vi "Bertta_v09_7.vi"() -> ()   [LabVIEW 2015]
panel:
  out "element":bool
  out "Started:":string
  in  "SHUTDOWN":bool
  in  "MASTER CONTROL":bool
  in  "Tab Control":T1(tab)
  in  "Read Seq":bool
  in  "Save Seq":bool
  in  "Configuration file":path=path "C:/Users/shresplab/Desktop/BerttaConfiguration.lvm" caption="Filename"
  in  "OK Button 2":bool
  out "Boolean":bool
  in  "User (initials)":string
  in  "Project name":string
  in  "Description":string
  out "Output file":string
  out "PUMP1":bool
  out "Target amount":dbl
  out "Scale weight":dbl
  out "Amount now":dbl
  out "Flow rate":dbl
  out "Time to target":dbl format="%<%H:%M:%S>t"
  out "Current step":dbl
  out "Target":dbl
  out "Amount now":dbl
  out "Amount now":dbl
  out "Target":dbl
  out "Current step":dbl
  out "Time to target":dbl format="%<%H:%M:%S>t"
  out "Flow rate":dbl
  out "Amount now":dbl
  out "Scale weight":dbl
  out "Target amount":dbl
  out "PUMP2":bool
  out "Sensor OK 6":bool
  out "Sensor OK 5":bool
  out "Sensor OK 4":bool
  out "Sensor OK 3":bool
  in  "OK Button":bool
  in  "Add comment":string
  out "PUMP3":bool
  out "Target amount":dbl
  out "Scale weight":dbl
  out "Amount now":dbl
  out "Flow rate":dbl
  out "Time to target":dbl format="%<%H:%M:%S>t"
  out "Current step":dbl
  out "Target":dbl
  out "Amount now":dbl
  out "Tr":dbl
  out "Tj in":dbl
  out "Tj out":dbl
  out "T set":dbl
  out "Current step":i32
  out "RPM":dbl
  out "Torque 2":dbl
  out "Waveform Chart 5":dynamicdata(graph)
  out "Waveform Chart 6":dynamicdata(graph)
  out "Waveform Chart 7":dynamicdata(graph)
  in  "Tab Control 2":T2(tab)
  out "Waveform Chart 3":dynamicdata(graph)
  out "Waveform Chart 8":dynamicdata(graph)
  out "Waveform Chart 11":dynamicdata(graph)
  out "Waveform Chart 13":dynamicdata(graph)
  out "Waveform Chart 9":dynamicdata(graph)
  out "Table":string[][](table)=[["14.8.2017 18.06.59", "0,000000", "417,670000", "-0,150000", "1,000000", "22,220000", "23,366837", "23,574959", "23,985852", "23,690000", "240,000000", "4,000000", "0,000000", "397,000000", "-397,000000", "1,000000"], ["14.8.2017 18.07.06", "0,000000", "417,640000", "-0,120000", "1,000000", "22,220000", "23,763115", "23,906257", "23,985694", "23,680000", "240,000000", "4,000000", "0,000000", "397,000000", "-397,000000", "1,000000"], ["14.8.2017 18.07.13", "0,000000", "417,640000", "-0,120000", "1,000000", "22,220000", "23,965922", "24,013440", "23,984906", "23,670000", "240,000000", "4,100000", "3,000000", "397,000000", "-397,000000", "1,000000"], ["14.8.2017 18.07.21", "0,000000", "417,640000", "-0,120000", "1,000000", "22,220000", "23,943860", "23,900110", "23,987113", "23,670000", "240,000000", "4,000000", "0,000000", "397,000000", "-397,000000", "1,000000"], ["14.8.2017 18.07.28", "0,000000", "417,640000", "-0,120000", "1,000000", "22,220000", "23,736328", "23,600018", "23,989004", "23,660000", "240,000000", "4,000000", "0,000000", "397,000000", "-397,000000", "1,000000"], ["14.8.2017 18.07.36", "0,000000", "417,640000", "-0,120000", "1,000000", "22,220000", "23,480910", "23,324538", "23,991053", "23,660000", "240,000000", "4,000000", "0,000000", "397,000000", "-397,000000", "1,000000"], ["14.8.2017 18.07.43", "0,000000", "417,640000", "-0,120000", "2,000000", "22,220000", "23,195579", "23,008270", "23,999093", "23,650000", "240,000000", "4,000000", "0,000000", "397,000000", "-397,000000", "1,000000"], ["14.8.2017 18.07.51", "0,000000", "417,650000", "-417,650000", "1,000000", "22,220000", "22,862541", "22,649021", "24,003979", "23,650000", "240,000000", "4,000000", "0,000000", "397,000000", "-397,000000", "2,000000"], ["14.8.2017 18.07.58", "0,000000", "417,640000", "0,010000", "1,000000", "22,220000", "22,541353", "22,354878", "24,005398", "23,650000", "240,000000", "4,000000", "0,000000", "397,000000", "-397,000000", "1,000000"], ["14.8.2017 18.08.06", "0,000000", "417,640000", "0,010000", "1,000000", "22,220000", "22,347931", "22,253738", "24,007605", "23,640000", "240,000000", "4,100000", "0,000000", "397,000000", "-397,000000", "1,000000"], ["14.8.2017 18.08.13", "0,000000", "417,640000", "0,010000", "1,000000", "22,220000", "22,329030", "22,302102", "24,006028", "23,640000", "240,000000", "4,000000", "0,000000", "395,820000", "-395,820000", "1,000000"], ["14.8.2017 18.08.20", "0,000000", "417,640000", "0,010000", "1,000000", "22,220000", "22,466849", "22,511320", "24,002403", "23,630000", "240,000000", "4,000000", "0,000000", "395,830000", "-0,010000", "1,000000"], ["14.8.2017 18.08.28", "0,000000", "417,640000", "0,010000", "1,000000", "22,220000", "22,707062", "22,835101", "24,000984", "23,620000", "240,000000", "4,000000", "0,000000", "395,830000", "-0,010000", "1,000000"], ["14.8.2017 18.08.35", "0,000000", "417,640000", "0,010000", "1,000000", "22,220000", "23,054104", "23,232979", "24,001299", "23,600000", "240,000000", "4,000000", "0,000000", "395,830000", "-0,010000", "1,000000"], ["14.8.2017 18.08.43", "0,000000", "417,640000", "0,010000", "1,000000", "22,220000", "23,412371", "23,522793", "24,002560", "23,590000", "240,000000", "4,000000", "0,000000", "395,820000", "0,000000", "1,000000"], ["14.8.2017 18.08.51", "0,000000", "417,640000", "0,010000", "1,000000", "22,220000", "23,596247", "23,656125", "24,003821", "23,580000", "240,000000", "4,000000", "0,000000", "395,820000", "0,000000", "1,000000"]]
  in  "Reset":bool
  in  "Numeric 4":dbl=20.0
  in  "Numeric 3":dbl=30.0
  in  "Numeric 2":dbl=40.0
  in  "Numeric 1":dbl=30.0
  in  "Numeric":dbl=20.0
  out "Boolean 12":bool
  out "Boolean 7":bool
  out "Boolean 6":bool
  out "Boolean 5":bool
  out "Boolean 4":bool
  out "Boolean 19":bool
  in  "Numeric 5":dbl=5.0
  in  "Numeric 6":dbl=5.0
  in  "Numeric 7":dbl=5.0
  in  "Numeric 8":dbl=5.0
  in  "T ext / T ext 2":enum32{"External 1", "External 2"}(radio)
  out "Sensor OK":bool
  in  "T fail":dbl=20.0
  in  "?":bool
  in  "T manual setpoint":dbl=20.0
  in  "Lauda port":dbl=9.0
  in  "Manual select":enum32{"Tr", "Tj"}(radio)
  in  "PAUSE":bool
  out "Waveform Chart":dynamicdata(graph)
  out "T external 2":dbl
  out "Led11 5":bool
  in  "Port":i32=10
  in  "Radio Buttons 4":enum32{"Reglo Digital", "Reglo Analog", "PAM"}(radio)
  out "Speed":dbl
  out "mA":dbl format="%#_2g"
  in  "Port":i32=16
  out "RPM":dbl format="%_4f"
  out "Led10 3":bool
  out "Led9 3":bool
  out "Led8 3":bool
  out "Led7 3":bool
  out "Led6 3":bool
  out "Led5 3":bool
  out "Led4 3":bool
  out "Led3 3":bool
  out "Led2 3":bool
  out "Led1 3":bool
  in  "PumpSeq 4":dbl[][](array[numeric])=[[1.0, 2.0, 0.0], [2.0, 2.0, 0.0], [3.0, 2.0, 0.0], [0.0, 0.0, 0.0], [0.0, 0.0, 0.0], [0.0, 0.0, 0.0], [0.0, 0.0, 0.0], [0.0, 0.0, 0.0], [0.0, 0.0, 0.0], [0.0, 0.0, 0.0], [0.0, 1.0, 0.0]]
  in  "?":bool
  out "Flow rate (g/min)":dbl
  out "Scale reading":dbl
  out "Step amount now":dbl
  in  "Grams / min":dbl
  out "Waveform Chart 14":dynamicdata(graph)
  in  "?":bool
  out "Total amount now":dbl
  out "Led11 4":bool
  in  "Reset 5":bool
  out "Elapsed / step":i32
  out "Time to target":dbl format="%<%H:%M:%S>t"
  out "Led11":bool
  in  "Port":i32=11
  in  "Radio Buttons 2":enum32{"Reglo Digital", "Reglo Analog", "PAM"}(radio)
  out "Speed":dbl
  out "mA":dbl format="%#_2g"
  in  "Port":i32=15
  out "RPM":dbl format="%_4f"
  out "Led10":bool
  out "Led9":bool
  out "Led8":bool
  out "Led7":bool
  out "Led6":bool
  out "Led5":bool
  out "Led4":bool
  out "Led3":bool
  out "Led2":bool
  out "Led1":bool
  in  "PumpSeq 2":dbl[][](array[numeric])=[[1.0, 1.0, 7.0], [2.0, 1.0, 2.0], [3.0, 1.0, 100.0], [0.0, 0.0, 0.0], [0.0, 0.0, 0.0], [0.0, 0.0, 0.0], [0.0, 0.0, 0.0], [0.0, 0.0, 0.0], [0.0, 0.0, 0.0], [0.0, 0.0, 0.0], [0.0, 1.0, 0.0]]
  in  "?":bool
  out "Flow rate (g/min)":dbl
  out "Scale reading":dbl
  out "Step amount now":dbl
  in  "Grams / min":dbl
  out "Waveform Chart 10":dynamicdata(graph)
  in  "?":bool
  out "Total amount now":dbl
  out "Led11":bool
  in  "Reset 3":bool
  out "Elapsed / step":i32
  out "Time to target":dbl format="%<%H:%M:%S>t"
  out "Led11 3":bool
  in  "Port":i32=12
  in  "Radio Buttons 3":enum32{"Reglo Digital", "Reglo Analog", "PAM"}(radio)
  out "Speed":dbl
  out "mA":dbl format="%#_2g"
  in  "Port":i32=14
  out "RPM":dbl format="%_4f"
  out "Led10 2":bool
  out "Led9 2":bool
  out "Led8 2":bool
  out "Led7 2":bool
  out "Led6 2":bool
  out "Led5 2":bool
  out "Led4 2":bool
  out "Led3 2":bool
  out "Led2 2":bool
  out "Led1 2":bool
  in  "PumpSeq 3":dbl[][](array[numeric])=[[1.0, 1.0, 7.0], [2.0, 1.0, 2.0], [3.0, 1.0, 100.0], [0.0, 0.0, 0.0], [0.0, 0.0, 0.0], [0.0, 0.0, 0.0], [0.0, 0.0, 0.0], [0.0, 0.0, 0.0], [0.0, 0.0, 0.0], [0.0, 0.0, 0.0], [0.0, 1.0, 0.0]]
  in  "?":bool
  out "Flow rate (g/min)":dbl
  out "Scale reading":dbl
  out "Step amount now":dbl
  in  "Grams / min":dbl
  out "Waveform Chart 12":dynamicdata(graph)
  in  "?":bool
  out "Total amount now":dbl
  out "Led11 2":bool
  in  "Reset 4":bool
  out "Elapsed / step":i32
  out "Time to target":dbl format="%<%H:%M:%S>t"
  in  "Bypass select 2":enum32{"Remote", "Manual"}(radio)=enum."Manual"
  in  "Port":dbl=13.0
  out "RPM":dbl
  out "Torque":dbl
  in  "Set RPM":dbl(slide) scale=0.0..2000.0
  out "Waveform Chart 4":dynamicdata(graph)
  in  "Treshold (T/C)":dbl=0.5
  out "DAQ 9217 (PT100)":errorcluster
  out "Config File":dbl[][](array[numeric])
  # "Temperature sensor:"
  # "Manual control:"
  # "PUMP & SCALE 1"
  # "STEP"
  # "TOTAL"
  # "PUMP & SCALE 2"
  # "STEP"
  # "TOTAL"
  # "PUMP & SCALE 3"
  # "STEP"
  # "TOTAL"
  # "Manual control"
  # "Secondary temperature sensor"
  # "Device communication"
  # "Temp"
  # "Time"
  # "Grams    /   min"
  # "End of sequence"
  # "Manual control"
  # "Device communication"
  # "Pump configuration"
  # "Scale configuration"
  # "SCALE 1"
  # "Grams    /   min"
  # "End of sequence"
  # "Manual control"
  # "Device communication"
  # "Pump configuration"
  # "Scale configuration"
  # "SCALE 2"
  # "Grams    /   min"
  # "End of sequence"
  # "Manual control"
  # "Device communication"
  # "Pump configuration"
  # "Scale configuration"
  # "SCALE 3"
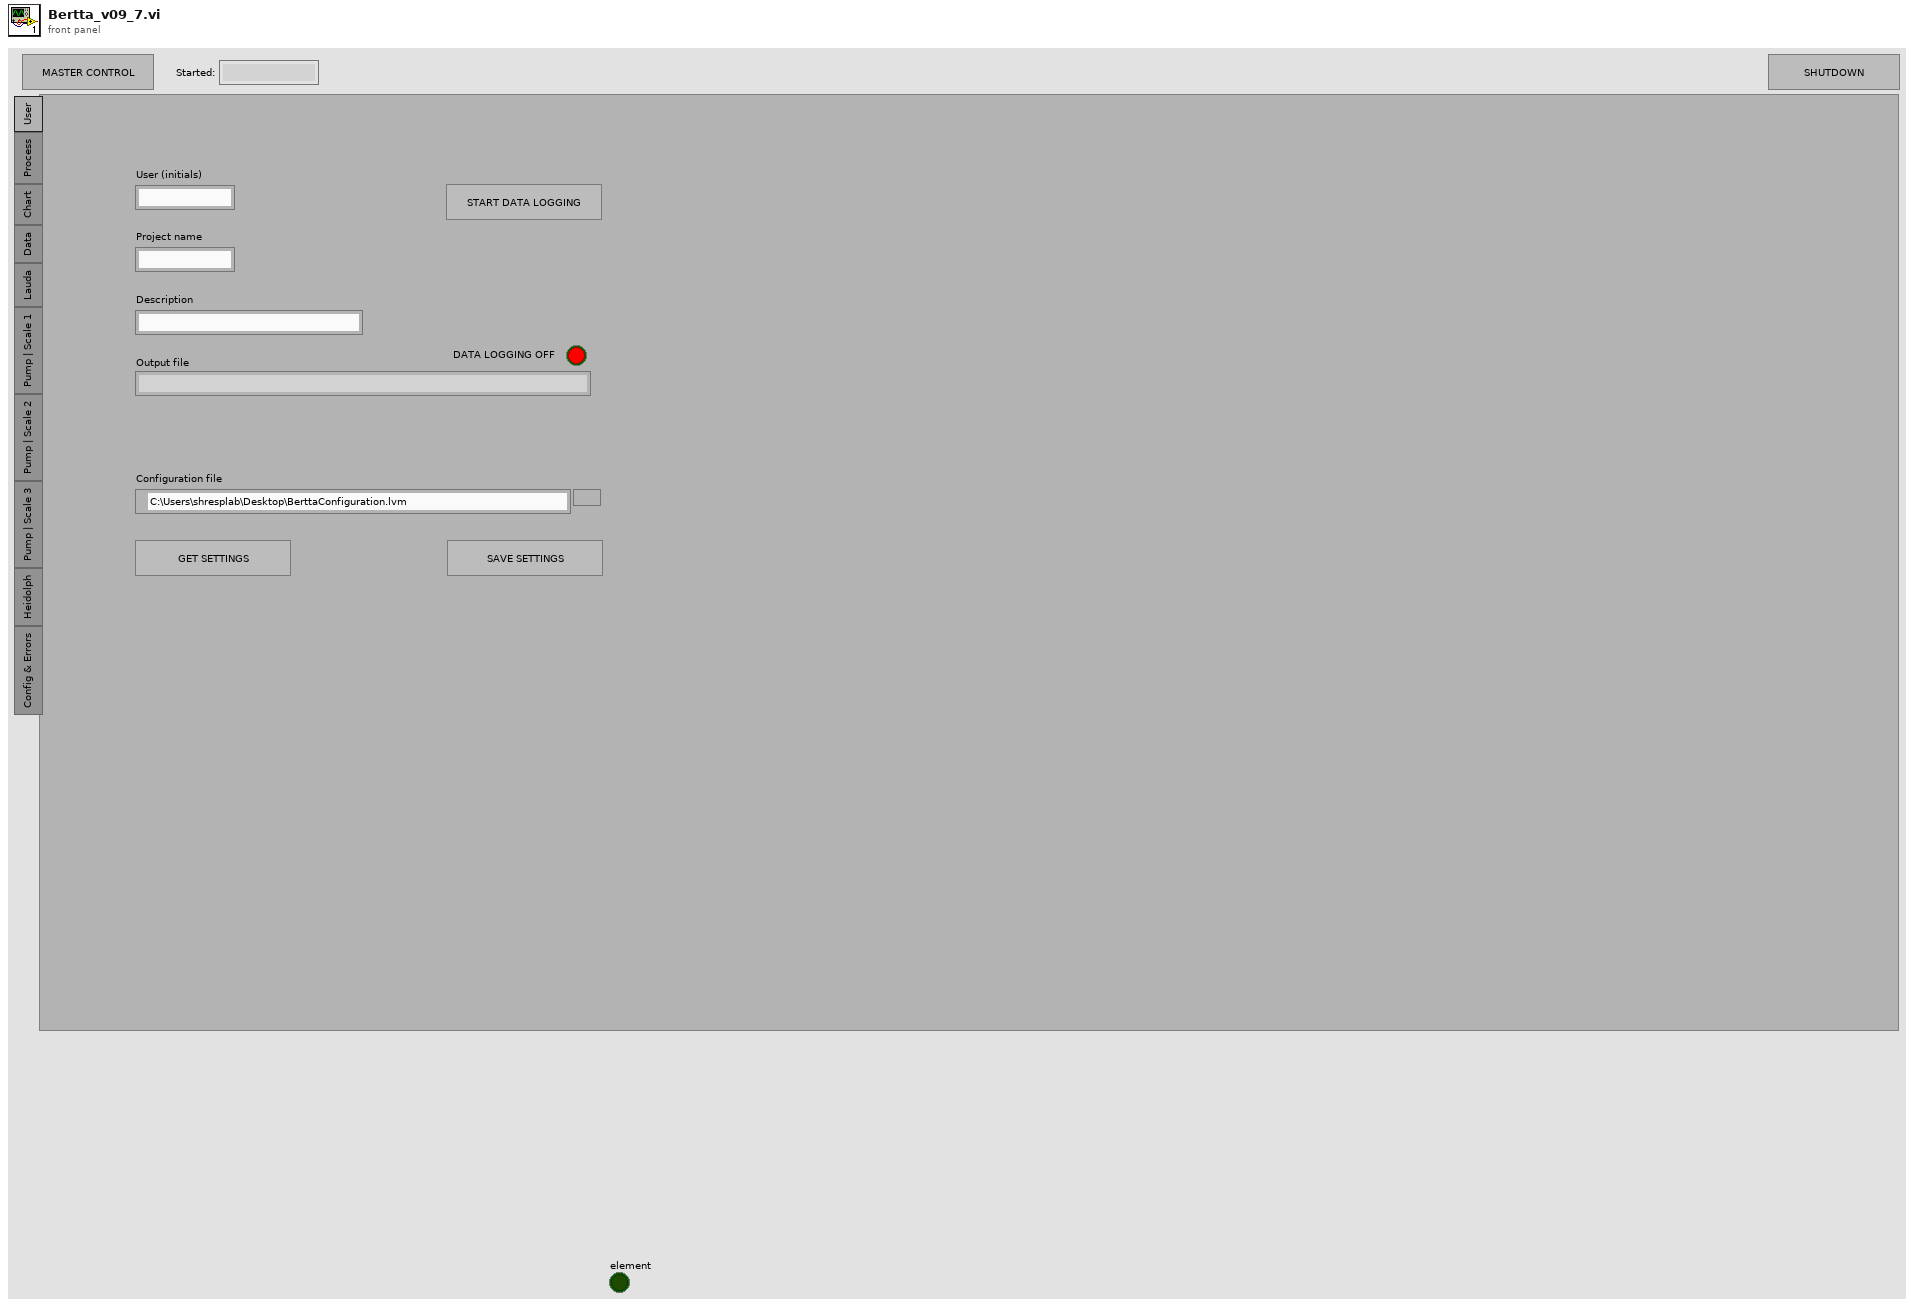
[diagram p1: front panel]
types:
  T1 = enum32{"User", "Process", "Chart", "Data", "Lauda", "Pump | Scale 1", "Pump | Scale 2", "Pump | Scale 3", "Heidolph", "Config & Errors"}
  T2 = enum32{"Temperatures", "Scale / Pump 1", "Scale / Pump 2", "Scale / Pump 3", "RPM / torque"}
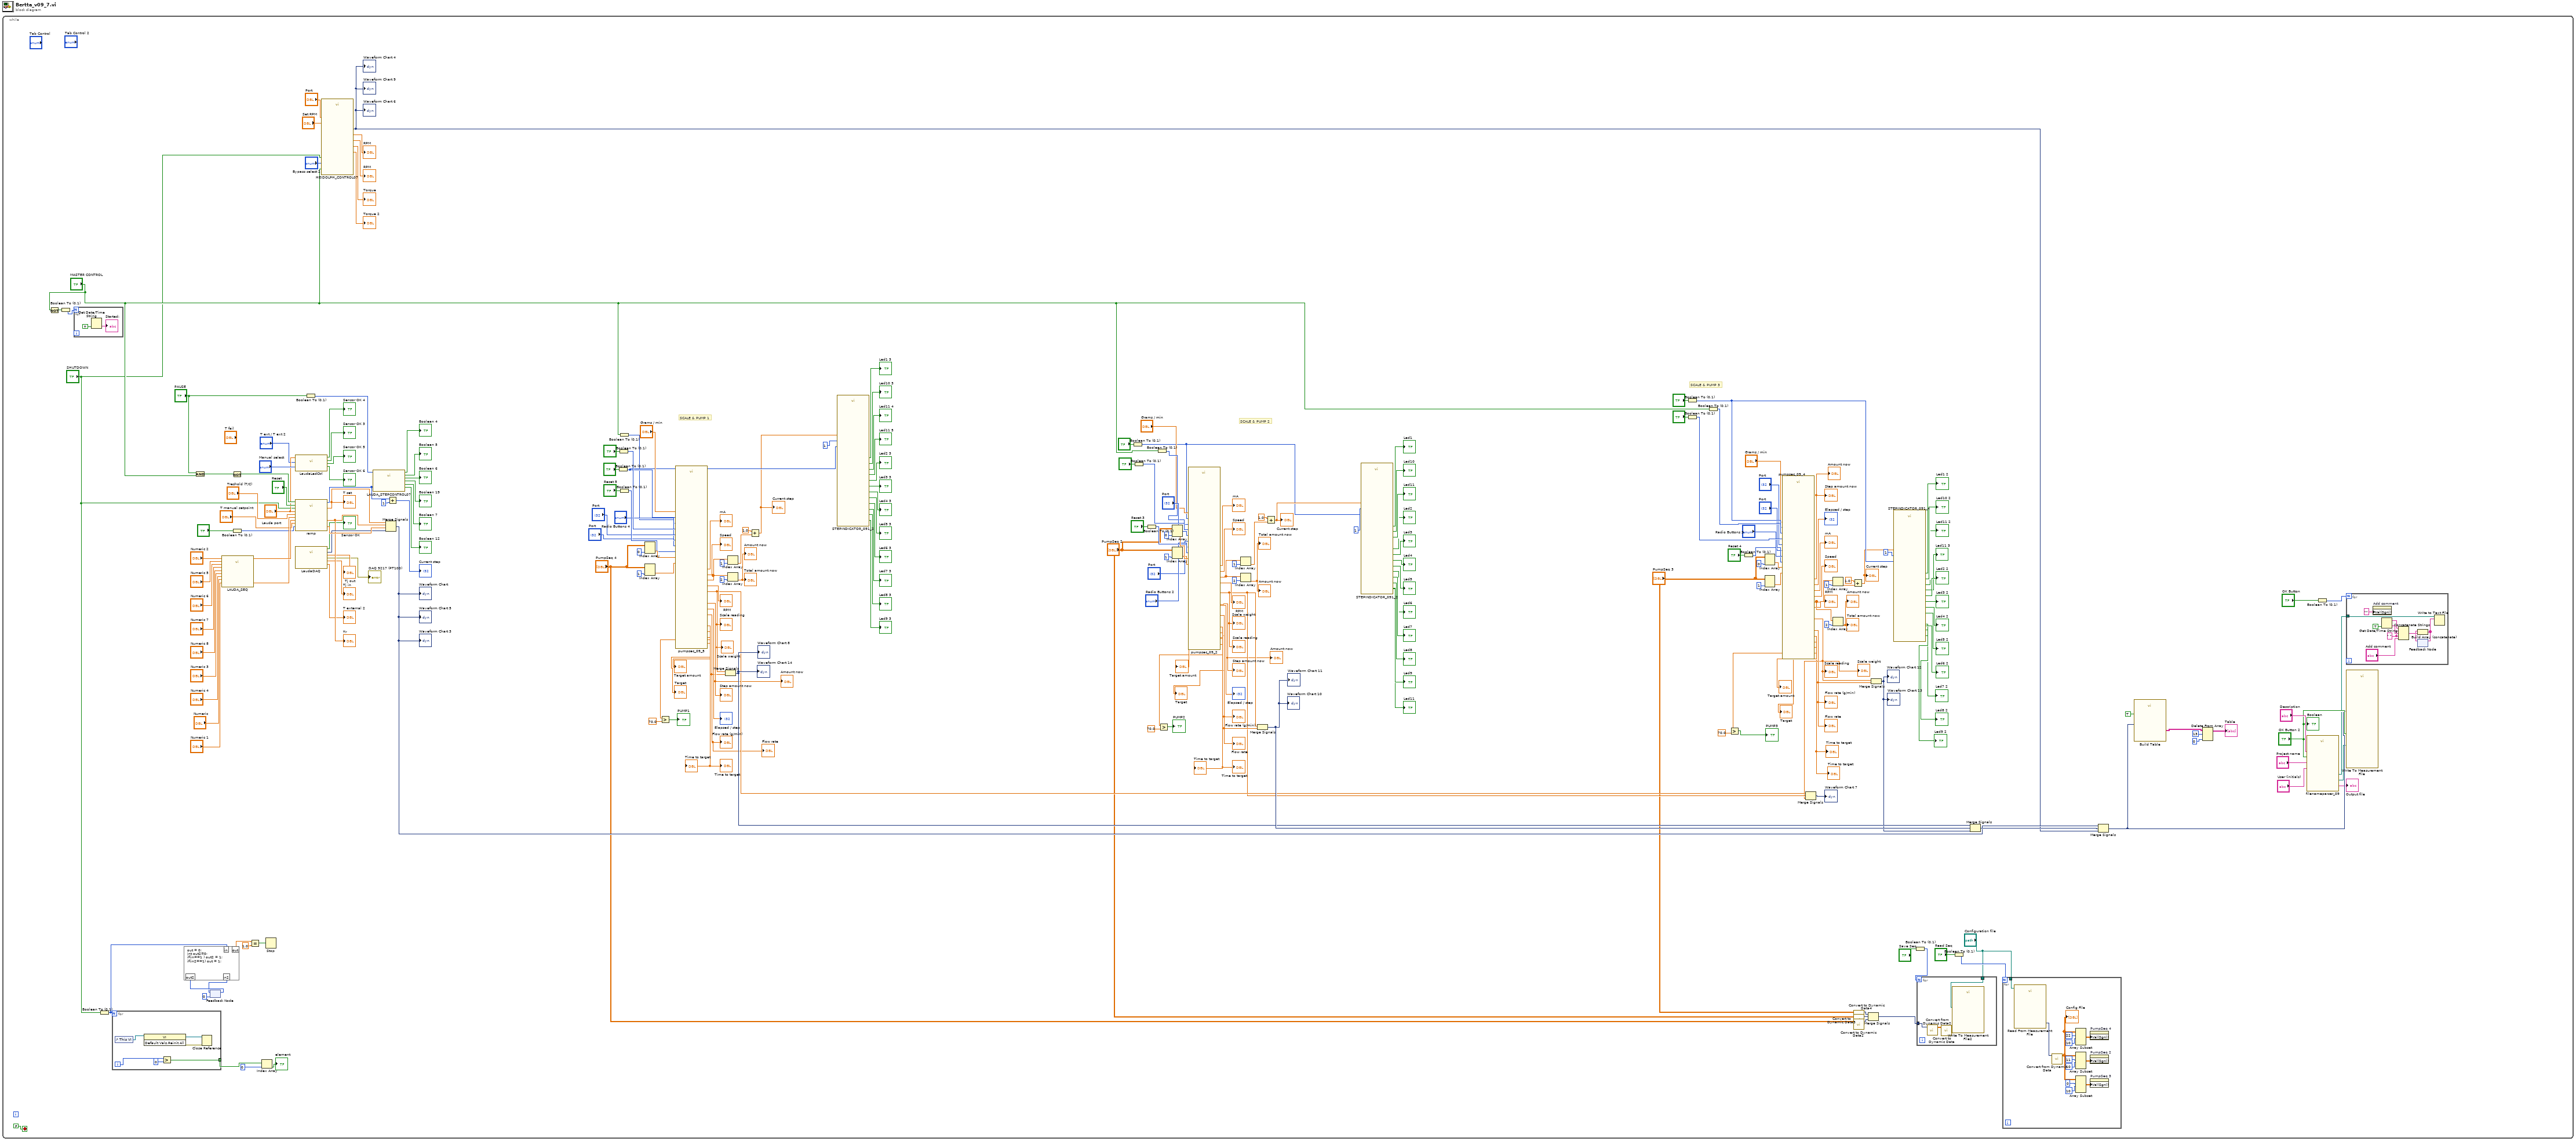
[diagram p0: block diagram]
diagram:
  n1 = while {
    stop <- FALSE stop-if-true
    # "SCALE & PUMP 1"
    # "SCALE & PUMP 3"
    # "SCALE & PUMP 2"
    n2 = Not(x="MASTER CONTROL") -> (.not. x?=w228:bool)
    n3 = Boolean To (0,1)(Boolean=w228) -> (0, 1=w229:i16)
    n4 = for {
      N: w229 -> [_]
      n5 = Get Date/Time String(want seconds? (F)=TRUE) -> (time string=→"Started:":string)  [unwired: 2 in, 1 out]
    }
    n6 = Boolean To (0,1)(Boolean="SHUTDOWN") -> (0, 1=w206:i16)
    n7 = for {
      N: w206 -> [_]
      tunnel: [w272] -> w227 mode=indexing
      i -> [w274]
      n8 = control-ref of="This VI"() -> (w277:refnum<vi>)
      n9 = invoke class="VI" method="Default Vals.Reinit All"(reference=w277) -> (reference out=w275:refnum<vi>, error out=w276:errorcluster)  [unwired: 2 in, 1 out]
      n10 = Greater?(x=w274, y=0) -> (0:w272:bool)
      n11 = Close Reference(reference=w275, error in (no error)=w276) -> ()  [unwired: 1 out]
    }
    n12 = And(x="PAUSE", y="MASTER CONTROL") -> (x .and. y?=w161:bool)
    n13 = feedback #1(0) -> (w204:i32)
    n14 = formula code="out = 0;\nint out2=0;\nif(in==1 ) out2 = 1;\nif(in2==1) out = 1;"("in"=w206, "in2"=w204) -> ("out"=w208:dbl, "out2"=w205:i32)
    n15 = feedback-in #1(w205) -> ()
    n16 = call "LAUDA_SEQ.vi"("Numeric 2"="Numeric 2", "Numeric 1"="Numeric 1", "Numeric"="Numeric", "Numeric 5"="Numeric 5", "Numeric 6"="Numeric 6", "Numeric 7"="Numeric 7", "Numeric 8"="Numeric 8", "Numeric 3"="Numeric 3", "Numeric 4"="Numeric 4") -> ("output array"=w149:dbl[], "output array 2"=w148:dbl[])  [unwired: 5 in]
    n17 = Not(x=w161) -> (.not. x?=w160:bool)
    n18 = Boolean To (0,1)(Boolean="?") -> (0, 1=w146:i16)
    n19 = Equal?(x=w208, y=1.0) -> (x = y?=w207:bool)
    n20 = Index Array(array=w227, index=0) -> (element=→"element":bool)
    n21 = Stop(stop? (T)=w207) -> ()
    n22 = call "LaudaLedCtrl.vi"("Manual select"="Manual select", "T ext / T ext in"="T ext / T ext 2", "Lauda port"="Lauda port") -> ("Sensor OK 5"=→"Sensor OK 5":bool, "Sensor OK 3"=→"Sensor OK 3":bool, "Sensor OK 4"=→"Sensor OK 4":bool, "Sensor OK 6"=→"Sensor OK 6":bool)  [unwired: 5 in]
    n23 = call "ramp.vi"("pause"=w160, "manual"=w146, "T_man"="T manual setpoint", "Seq"=w149, "reset"="Reset", "TimeParams"=w148, "shutdown"="SHUTDOWN", "port"="Lauda port", "treshold"="Treshold (T/C)") -> ("T in"=w55:dbl, "STEP"=w23:i32, "T ext"=w41:dbl, "T control"=w42:dbl)  [unwired: 2 in, 1 out]
    "Tr" <- w41
    "T set" <- w42
    n24 = call "LaudaDAQ.vi"() -> ("error out"=→"DAQ 9217 (PT100)":errorcluster, 1:"Tj out"=→"Tj out":dbl, "data"=w54:dynamicdata, "Sensor OK"=→"Sensor OK":bool, 4:"Tj out"=→"Tj in":dbl, "T external 2"=→"T external 2":dbl)  [unwired: 6 in]
    n25 = Boolean To (0,1)(Boolean="PAUSE") -> (0, 1=w201:i16)
    n26 = call "HEIDOLPH_CONTROL07.vi"("master"="MASTER CONTROL", "shutdown"="SHUTDOWN", "Bypass select"="Bypass select 2", "Set RPM"="Set RPM", "Device port"="Port") -> ("Dynamic Data"=w56:dynamicdata, "RPM"=→"RPM":dbl, "RPM 2"=→"RPM":dbl, "Torque"=→"Torque":dbl, "Torque 2"=→"Torque 2":dbl)  [unwired: 2 in]
    "Waveform Chart 4" <- w56
    "Waveform Chart 6" <- w56
    "Waveform Chart 9" <- w56
    n27 = call "LAUDA_STEPCONTROL07.vi"("step"=w23, "pause"=w201) -> ("Boolean 13"=→"Boolean 19":bool, "Boolean 6"=→"Boolean 6":bool, "Boolean 5"=→"Boolean 5":bool, "Boolean 4"=→"Boolean 4":bool, "Boolean 7"=→"Boolean 7":bool, "Boolean 12"=→"Boolean 12":bool)  [unwired: 4 in]
    n28 = Merge Signals(w42, w41, w55, w54) -> (w57:dynamicdata)
    "Waveform Chart 3" <- w57
    "Waveform Chart" <- w57
    "Waveform Chart 5" <- w57
    n29 = Add(x=w23, y=1) -> (x+y=→"Current step":i32)
    n30 = Boolean To (0,1)(Boolean="?") -> (0, 1=w66:i16)
    n31 = Boolean To (0,1)(Boolean="?") -> (0, 1=w76:i16)
    n32 = Boolean To (0,1)(Boolean="MASTER CONTROL") -> (0, 1=w62:i16)
    n33 = Boolean To (0,1)(Boolean="Reset 5") -> (0, 1=w75:i16)
    n34 = Index Array(array="PumpSeq 4", index (col)=0) -> (element=w80:dbl[])  [unwired: 1 in]
    n35 = Index Array(array="PumpSeq 4", index (col)=1) -> (element=w101:dbl[])  [unwired: 1 in]
    n36 = call "pumpsec_09_5.vi"("reset"=w75, "master"=w62, "manual"=w66, "pause"=w76, "Port"="Port", "pump_type"="Radio Buttons 4", "port, Reglo D"="Port", "Target"=w80, "fr_manual"="Grams / min", "Time"=w101) -> ("pumpCtrl"=w36:dbl, "totaltarget"=→"Target":dbl, "target_step"=→"Target amount":dbl, "time_to_target"=→"Time to target" →"Time to target":dbl, "step_fr"=w9:dbl, "amount_step"=→"Amount now" →"Step amount now":dbl, "Reglo D"=→"RPM":dbl, "Scale"=w50:dbl, "mA"=→"mA":dbl, "elapsed_step"=→"Elapsed / step":dbl, "params"=w98:dbl[], "PAM"=→"Speed":dbl)  [unwired: 4 in, 2 out]
    "Flow rate" <- w9
    "Scale weight" <- w50
    "Scale reading" <- w50
    "Flow rate (g/min)" <- w9
    n37 = Greater?(x=w36, y=70.0) -> (0:→"PUMP1":bool)
    n38 = Merge Signals(w50, w9) -> (w60:dynamicdata)
    "Waveform Chart 8" <- w60
    "Waveform Chart 14" <- w60
    n39 = Index Array(array=w98, index=1) -> (element=w95:dbl)
    n40 = Index Array(array=w98, index=2) -> (element=→"Amount now" →"Total amount now":dbl)
    n41 = Add(x=1.0, y=w95) -> (x+y=w10:dbl)
    "Current step" <- w10
    n42 = call "STEPINDICATOR_091_2.vi"("current step"=w10, "enable"=i16 1, "manual"=w66) -> ("Led 8"=→"Led8 3":bool, "Led 10"=→"Led10 3":bool, "Led 11"=→"Led11 4":bool, "Led 7"=→"Led7 3":bool, "Led 1"=→"Led1 3":bool, "Led 6"=→"Led6 3":bool, "Led 2"=→"Led2 3":bool, "Led 12"=→"Led11 5":bool, "Led 5"=→"Led5 3":bool, "Led 4"=→"Led4 3":bool, "Led 3"=→"Led3 3":bool, "Led 9"=→"Led9 3":bool)  [unwired: 1 in]
    n43 = Boolean To (0,1)(Boolean="?") -> (0, 1=w141:i16)
    n44 = Boolean To (0,1)(Boolean="?") -> (0, 1=w194:i16)
    n45 = Boolean To (0,1)(Boolean="Reset 3") -> (0, 1=w191:i16)
    n46 = Boolean To (0,1)(Boolean="MASTER CONTROL") -> (0, 1=w185:i16)
    n47 = Index Array(array="PumpSeq 2", index (col)=0 ("disabled index (col)")) -> (element=w197:dbl[])  [unwired: 1 in]
    n48 = Index Array(array="PumpSeq 2", index (col)=1 ("disabled index (col)")) -> (element=w196:dbl[])  [unwired: 1 in]
    n49 = call "pumpsec_09_2.vi"("reset"=w191, "master"=w185, "manual"=w141, "pause"=w194, "Port"="Port", "pump_type"="Radio Buttons 2", "port, Reglo D"="Port", "Target"=w197, "fr_manual"="Grams / min", "Time"=w196) -> ("pumpCtrl"=w32:dbl, "totaltarget"=→"Target":dbl, "target_step"=→"Target amount":dbl, "time_to_target"=→"Time to target" →"Time to target":dbl, "step_fr"=w53:dbl, "amount_step"=→"Amount now" →"Step amount now":dbl, "Reglo D"=→"RPM":dbl, "Scale"=w49:dbl, "mA"=→"mA":dbl, "elapsed_step"=→"Elapsed / step":dbl, "params"=w186:dbl[], "PAM"=→"Speed":dbl)  [unwired: 4 in, 2 out]
    "Scale weight" <- w49
    "Flow rate" <- w53
    "Scale reading" <- w49
    "Flow rate (g/min)" <- w53
    n50 = Greater?(x=w32, y=70.0) -> (0:→"PUMP2":bool)
    n51 = Index Array(array=w186, index=1) -> (element=w189:dbl)
    n52 = Index Array(array=w186, index=2) -> (element=→"Amount now" →"Total amount now":dbl)
    n53 = Merge Signals(w49, w53) -> (w63:dynamicdata)
    "Waveform Chart 11" <- w63
    "Waveform Chart 10" <- w63
    n54 = Add(x=1.0, y=w189) -> (x+y=w179:dbl)
    "Current step" <- w179
    n55 = call "STEPINDICATOR_091_2.vi"("current step"=w179, "enable"=i16 1, "manual"=w141) -> ("Led 8"=→"Led8":bool, "Led 10"=→"Led10":bool, "Led 11"=→"Led11":bool, "Led 7"=→"Led7":bool, "Led 1"=→"Led1":bool, "Led 6"=→"Led6":bool, "Led 2"=→"Led2":bool, "Led 12"=→"Led11":bool, "Led 5"=→"Led5":bool, "Led 4"=→"Led4":bool, "Led 3"=→"Led3":bool, "Led 9"=→"Led9":bool)  [unwired: 1 in]
    n56 = Boolean To (0,1)(Boolean="?") -> (0, 1=w135:i16)
    n57 = Boolean To (0,1)(Boolean="?") -> (0, 1=w134:i16)
    n58 = Boolean To (0,1)(Boolean="MASTER CONTROL") -> (0, 1=w136:i16)
    n59 = Boolean To (0,1)(Boolean="Reset 4") -> (0, 1=w115:i16)
    n60 = Index Array(array="PumpSeq 3", index (col)=0 ("disabled index (col)")) -> (element=w118:dbl[])  [unwired: 1 in]
    n61 = Index Array(array="PumpSeq 3", index (col)=1 ("disabled index (col)")) -> (element=w117:dbl[])  [unwired: 1 in]
    n62 = call "pumpsec_09_4.vi"("reset"=w115, "master"=w136, "manual"=w135, "pause"=w134, "Port"="Port", "pump_type"="Radio Buttons 3", "port, Reglo D"="Port", "Target"=w118, "fr_manual"="Grams / min", "Time"=w117) -> ("pumpCtrl"=w29:dbl, "totaltarget"=→"Target":dbl, "target_step"=→"Target amount":dbl, "time_to_target"=→"Time to target" →"Time to target":dbl, "step_fr"=w52:dbl, "amount_step"=→"Amount now" →"Step amount now":dbl, "Reglo D"=→"RPM":dbl, "Scale"=w48:dbl, "mA"=→"mA":dbl, "elapsed_step"=→"Elapsed / step":dbl, "params"=w103:dbl[], "PAM"=→"Speed":dbl)  [unwired: 4 in, 2 out]
    "Scale weight" <- w48
    "Flow rate" <- w52
    "Scale reading" <- w48
    "Flow rate (g/min)" <- w52
    n63 = Greater?(x=w29, y=70.0) -> (0:→"PUMP3":bool)
    n64 = Merge Signals(w50, w49, w48) -> (→"Waveform Chart 7":dynamicdata)
    n65 = Index Array(array=w103, index=1) -> (element=w104:dbl)
    n66 = Index Array(array=w103, index=2) -> (element=→"Amount now" →"Total amount now":dbl)
    n67 = Add(x=1.0, y=w104) -> (x+y=w102:dbl)
    "Current step" <- w102
    n68 = call "Convert to Dynamic Data4"("2D Array"="PumpSeq 3") -> ("Dynamic Data Type"=w1:dynamicdata)  [unwired: 3 in]
    n69 = call "Convert to Dynamic Data3"("2D Array"="PumpSeq 2") -> ("Dynamic Data Type"=w3:dynamicdata)  [unwired: 3 in]
    n70 = call "Convert to Dynamic Data2"("2D Array"="PumpSeq 4") -> ("Dynamic Data Type"=w6:dynamicdata)  [unwired: 3 in]
    n71 = Merge Signals(w1, w3, w6) -> (w5:dynamicdata)
    n72 = Merge Signals(w48, w52) -> (w59:dynamicdata)
    "Waveform Chart 13" <- w59
    "Waveform Chart 12" <- w59
    n73 = call "STEPINDICATOR_091_4.vi"("current step"=w102, "enable"=i16 1, "manual"=w135) -> ("Led 8"=→"Led8 2":bool, "Led 10"=→"Led10 2":bool, "Led 11"=→"Led11 2":bool, "Led 7"=→"Led7 2":bool, "Led 1"=→"Led1 2":bool, "Led 6"=→"Led6 2":bool, "Led 2"=→"Led2 2":bool, "Led 12"=→"Led11 3":bool, "Led 5"=→"Led5 2":bool, "Led 4"=→"Led4 2":bool, "Led 3"=→"Led3 2":bool, "Led 9"=→"Led9 2":bool)  [unwired: 1 in]
    n74 = Boolean To (0,1)(Boolean="Save Seq") -> (0, 1=w225:i16)
    n75 = for {
      N: w225 -> [_]
      tunnel: w5 -> [w269]
      tunnel: "Configuration file" -> [w270]
      n76 = call "Convert from Dynamic Data2"("Dynamic Data Type"=w269) -> ("Array"=w268:dbl[][])  [unwired: 3 in]
      n77 = call "Convert to Dynamic Data"("2D Array"=w268) -> ("Dynamic Data Type"=w271:dynamicdata)  [unwired: 3 in]
      n78 = call "Write To Measurement File2"("Signals"=w271, "Filename"=w270) -> ()  [unwired: 15 in, 3 out]
    }
    n79 = Boolean To (0,1)(Boolean="Read Seq") -> (0, 1=w222:i16)
    n80 = Merge Signals(w60, w63, w59) -> (w58:dynamicdata)
    n81 = for {
      N: w222 -> [_]
      tunnel: "Configuration file" -> [w267]
      n82 = call "Read From Measurement File"("Filename"=w267) -> ("Signals"=w266:dynamicdata)  [unwired: 5 in, 5 out]
      n83 = call "Convert from Dynamic Data"("Dynamic Data Type"=w266) -> ("Array"=w258:dbl[][])  [unwired: 3 in]
      "Config File" <- w258
      n84 = Array Subset(array=w258, index (row)=22 ("index"), length (row)=10 ("length")) -> (w263:dbl[][])  [unwired: 2 in]
      n85 = Array Subset(array=w258, index (row)=11 ("index"), length (row)=10 ("length")) -> (w257:dbl[][])  [unwired: 2 in]
      n86 = Array Subset(array=w258, index (row)=0 ("index"), length (row)=10 ("length")) -> (w256:dbl[][])  [unwired: 2 in]
      n87 = property on="PumpSeq 4" class="Arr (strict)"("Val(Sgnl)"=w263) -> ()  [unwired: 2 in, 2 out]
      n88 = property on="PumpSeq 2" class="Arr (strict)"("Val(Sgnl)"=w257) -> ()  [unwired: 2 in, 2 out]
      n89 = property on="PumpSeq 3" class="Arr (strict)"("Val(Sgnl)"=w256) -> ()  [unwired: 2 in, 2 out]
    }
    n90 = Merge Signals(w57, w58, w56) -> (w218:dynamicdata)
    n91 = call "Build Table"("Include time data"=TRUE, "Signals"=w218) -> ("Table"=w217:string[][])  [unwired: 3 in, 6 out]
    n92 = Delete From Array(array=w217, length=13, index (col)=0 ("index (row)")) -> (array with subset deleted=→"Table":string[][])  [unwired: 1 in, 1 out]
    n93 = call "filenameparser_09.vi"("Description"="Description", "Project name"="Project name", "User (initials)"="User (initials)", "OK Button in"="OK Button 2") -> ("Output file"=→"Output file":string, "appended path 2"=w213:path, "appended path"=w212:path)  [unwired: 5 in]
    n94 = Boolean To (0,1)(Boolean="OK Button") -> (0, 1=w211:i16)
    n95 = for {
      N: w211 -> [_]
      tunnel: w212 -> [w248]
      w252 = " " ("string")
      n96 = property on="Add comment" class="Str"("Val(Sgnl)"="" ("Value (Signaling)")) -> ()  [unwired: 2 in, 2 out]
      n97 = Get Date/Time String(want seconds? (F)=TRUE) -> (date string=w255:string, time string=w253:string)  [unwired: 2 in]
      n98 = Concatenate Strings(w255, w252, w253, w252, "Add comment") -> (w251:string)
      n99 = feedback #2() -> (w250:string[])  [unwired: 1 in]
      n100 = Build Array (concatenate)(w250, w251) -> (w249:string[])
      n101 = feedback-in #2(w249) -> ()
      n102 = Write to Text File(file (use dialog)=w248, text=w249) -> ()  [unwired: 2 in, 3 out]
    }
    n103 = call "Write To Measurement File"("Signals"=w218, "Enable"="OK Button 2", "Filename"=w213) -> ()  [unwired: 14 in, 3 out]
    "Boolean" <- "OK Button 2"
  }
